vi "Actuator Channels 2 String Array.vi"(1 "Actuator Channels":T1) -> (0 "Array":string[](array[string]))   [LabVIEW 2013]
uses:
  Metadata/Actuator Channel Names.ctl
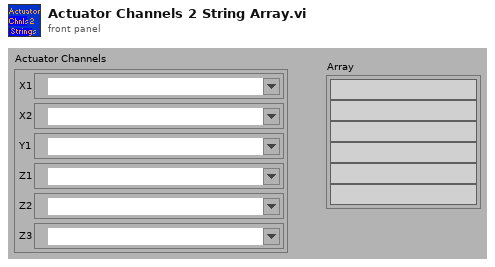
[diagram p1: front panel]
types:
  T1 = typedef "Actuator Channel Names.ctl" = cluster{"X1":refnum<k21>, "X2":refnum<k21>, "Y1":refnum<k21>, "Z1":refnum<k21>, "Z2":refnum<k21>, "Z3":refnum<k21>}
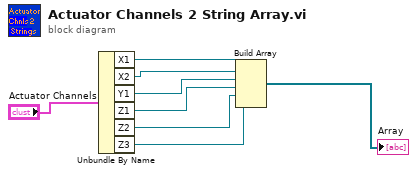
[diagram p0: block diagram]
diagram:
  n1 = Unbundle By Name("Actuator Channels") -> ("X1"=w2:refnum<k21>, "X2"=w3:refnum<k21>, "Y1"=w4:refnum<k21>, "Z1"=w5:refnum<k21>, "Z2"=w6:refnum<k21>, "Z3"=w7:refnum<k21>)
  n2 = Build Array(w2, w3, w4, w5, w6, w7) -> (→"Array":refnum<k21>[])
